vi "dll demo.vi"() -> ()   [LabVIEW 2024]
uses:
  Controls/calculate_doa_struct.ctl
  Controls/ant re&im.ctl
  Controls/Calc Para_int.ctl
  Controls/calculate_doa_head.ctl
  Controls/Calc Para_float.ctl
panel:
  out "calibration_parameters_radar":i32[](array[numeric])
  out "Result 2":bool
  in  "Boolean":bool
  out "arg1":sgl[](array[numeric])
  out "error out 2":errorcluster
  out "error out":errorcluster
  out "calibration_parameters":T1[](array[typedef])
  out "Result":bool
  in  "calculate_doa_head":T2={"frameID"=0, "waveID"=0, "TargetNum"=15, "InterNum"=0}
  out "Datas":T3[](array[typedef])
  in  "file (use dialog)":path=path "C:/Users/xsd/Desktop/data.txt"
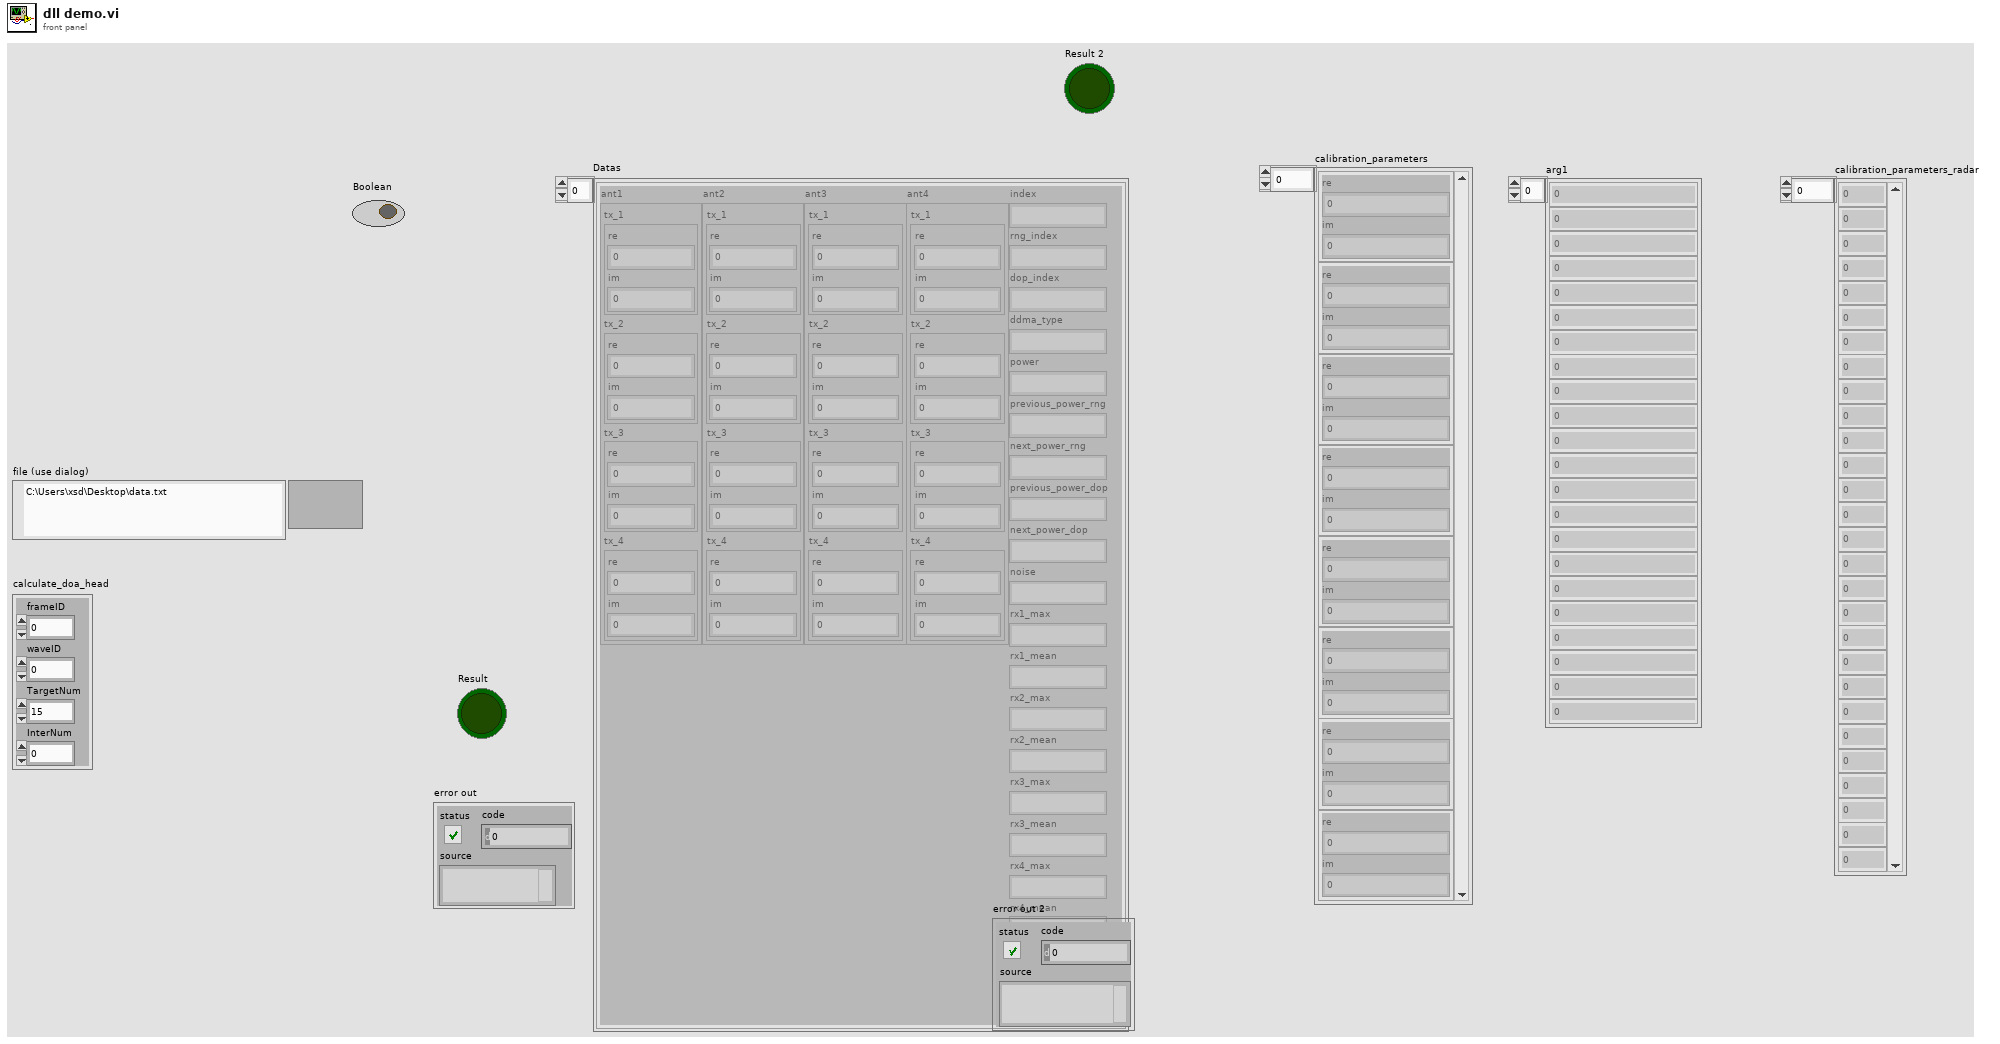
[diagram p1: front panel]
types:
  T1 = typedef "Calc Para_float.ctl" = cluster{"re":sgl, "im":sgl}
  T2 = typedef "calculate_doa_head.ctl" = cluster{"frameID":u16, "waveID":u16, "TargetNum":u16, "InterNum":u16}
  T3 = typedef "calculate_doa_struct.ctl" = cluster{"ant1":T4, "ant2":T4, "ant3":T4, "ant4":T4, "index":u16, "rng_index":u16, "dop_index":u16, "ddma_type":u16, "power":u32, "previous_power_rng":u32, "next_power_rng":u32, "previous_power_dop":u32, "next_power_dop":u32, "noise":u32, "rx1_max":u32, "rx1_mean":u32, "rx2_max":u32, "rx2_mean":u32, "rx3_max":u32, "rx3_mean":u32, "rx4_max":u32, "rx4_mean":u32, "reserved0":u32, "reserved1":u32}
  T4 = typedef "ant re&im.ctl" = cluster{"tx_1":T5, "tx_2":T5, "tx_3":T5, "tx_4":T5}
  T5 = typedef "Calc Para_int.ctl" = cluster{"re":i32, "im":i32}
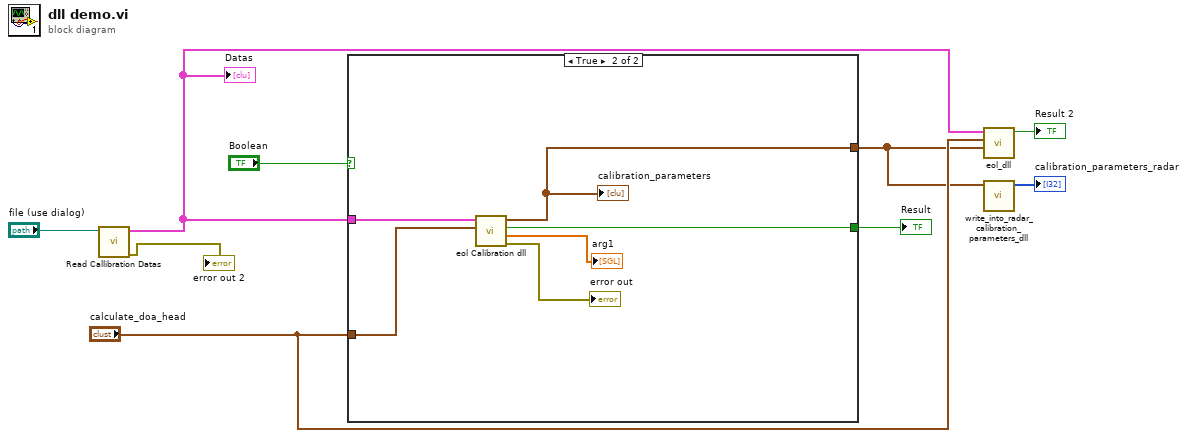
[diagram p0: block diagram]
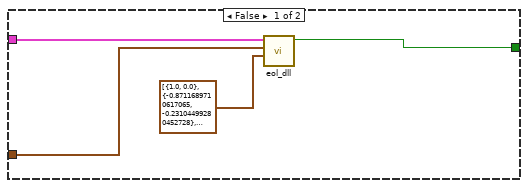
[diagram p2: hidden frame]
diagram:
  n1 = call "Read Callibration Datas.vi"("file (use dialog)"="file (use dialog)") -> ("error out"=→"error out 2":errorcluster, "Datas"=w4:T3[])  [unwired: 9 in]
  "Datas" <- w4
  n2 = case shown="True" "Boolean" {
    tunnel: w4 -> [w13 w19]
    tunnel: "calculate_doa_head" -> [w12 w18]
    tunnel: [w11 w15] -> w6
    tunnel: [_ w14] -> w1
    frame False {
      n3 = call "eol_dll.vi"("calibration_parameters"=T1[] [{"re"=1.0, "im"=0.0}, {"re"=-0.871169, "im"=-0.231045}, {"re"=0.279713, "im"=0.888431}, {"re"=0.690488, "im"=-0.833958}, {"re"=0.198737, "im"=0.917744}, {"re"=0.039368, "im"=-0.851752}, {"re"=-0.763411, "im"=0.433914}, {"re"=0.902014, "im"=0.46935}, {"re"=-0.69119, "im"=0.818481}, {"re"=0.792709, "im"=-0.555488}, {"re"=-0.921118, "im"=-0.392923}, {"re"=0.202966, "im"=1.142112}, {"re"=-0.160333, "im"=-1.795308}, {"re"=-0.276349, "im"=1.61779}, {"re"=1.569016, "im"=-0.635836}, {"re"=-1.606002, "im"=-1.118654}] ("Array"), "calculate_doa_head In"=w12, "Datas"=w13) -> ("Result"=w11:bool)  [unwired: 6 in, 2 out]
    }
    frame True {
      n4 = call "eol Calibration dll.vi"("calculate_doa_head"=w18, "calculate_doa_struct"=w19) -> ("error out"=→"error out":errorcluster, "arg1"=→"arg1":sgl[], "Result"=w15:bool, "calibration_parameters"=w14:T1[])  [unwired: 6 in]
      "calibration_parameters" <- w14
    }
  }
  "Result" <- w6
  n5 = call "eol_dll.vi"("calibration_parameters"=w1, "calculate_doa_head In"="calculate_doa_head", "Datas"=w4) -> ("Result"=→"Result 2":bool)  [unwired: 6 in, 2 out]
  n6 = call "write_into_radar_calibration_parameters_dll.vi"("calibration_parameters"=w1) -> ("calibration_parameters_radar"=→"calibration_parameters_radar":i32[])  [unwired: 8 in, 2 out]
